vi "Start SLSC FPGA.vi"(8 "error in (no error)":errorcluster, 11 "FPGA Ref in":refnum<k20>) -> (0 "error out":errorcluster)   [LabVIEW 2014, in "SLSC configuration Engine.lvlib"]
uses:
  SLSC configuration Engine.lvlib
  <vilib>/NI/LVFPGA Adv Session Resources/OpenByNameSubVI.vi
  Shared/Constants.vi
  <vilib>/rvi/interface/common/dynamic/niFpgaEscapeDelimiterAndNull.vi
  <vilib>/Utility/error.llb/Error Cluster From Error Code.vi
  <vilib>/rvi/errors/niLvFpgaAdjustHostInterfaceError.vi
  <vilib>/FPGAPlugInAG/Dynamic/niLvFpga_Close_Dynamic.vi
  <vilib>/NI/LVFPGA Adv Session Resources/OpenByName.xnode
  <vilib>/rvi/interface/nirviReadWriteControl/nirviReadWriteControl.xnode
  <vilib>/rvi/interface/nirviCloseFPGA/nirviCloseFPGA.xnode
  Shared/SLSC configuration Shared.lvlib
  NiFpgaLv.dll
  <vilib>/rvi/interface/Simulation/niFpgaSimulationCallBeginRW.vi
  <vilib>/NI/LVFPGA Adv Session Resources/LVFPGAAdvSessionResources.lvlib
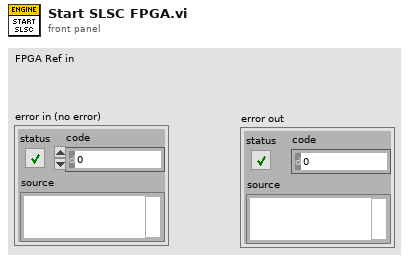
[diagram p1: front panel]
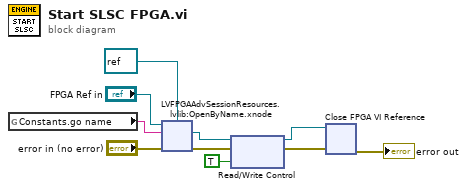
[diagram p0: block diagram]
diagram:
  n1 = global read "Constants.vi" "Constants.go name"() -> (w6:string)
  n2 = xnode "LVFPGAAdvSessionResources.lvlib:OpenByName.xnode"("FPGA VI Reference in"="FPGA Ref in", "Resource name in"=w6, "Single resource reference type in"=refnum<k20> refnum ("Single resource reference out"), "Error in"="error in (no error)") -> ("Single resource reference out"=w8:refnum<k20>, "Error out"=w10:errorcluster)  [unwired: 1 out]
  n3 = xnode "Read/Write Control"("FPGA VI Reference In"=w8, "error in"=w10, "Value"=TRUE) -> ("FPGA VI Reference Out"=w3:refnum<k20>, "error out"=w2:errorcluster)
  n4 = xnode "Close FPGA VI Reference"("FPGA VI Reference In"=w3, "error in"=w2) -> ("error out"=→"error out":errorcluster)
